vi "Basic Import Library.vi"(8 "Error In":errorcluster, 11 "system library name":string) -> (0 "Error Out":errorcluster, 3 "resulting string":string)   [LabVIEW 2014]
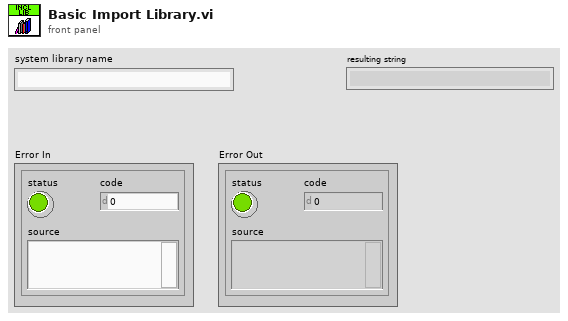
[diagram p1: front panel]
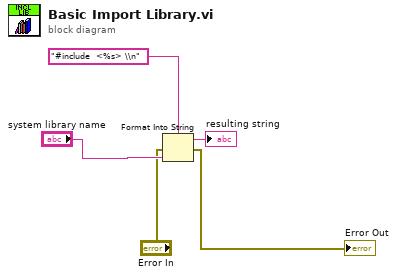
[diagram p0: block diagram]
diagram:
  n1 = Format Into String(format string="#include  <%s> \\n", error in="Error In", "system library name") -> (resulting string=→"resulting string":string, error out=→"Error Out":errorcluster)  [unwired: 1 in]
